vi "Send SetTemp Message.vi"(8 "error in (no error)":errorcluster, 10 "Cluster":cluster{"Temp":dbl, "Humid":dbl}, 11 "Execute":refnum<class "Execute.lvclass">) -> (0 "error out":errorcluster, 3 "Execute 2":refnum<class "Execute.lvclass">)   [LabVIEW 2018, in "QMH_Class.lvlib" / "TestManager.lvlib" / "SetTemp Message.lvclass"]
uses:
  SetTemp Message.lvclass
  Execute_class/Execute.lvclass
  E:/0 File/GITSync/DynoToolPlus/0 LabviewCode/0 Support/Message Queue_Class/Class/Message_class/InterfaceMessage/Interface Message.lvclass
  SetTemp Message.lvclass/SetTemp Message.ctl
  Execute_class/Execute.lvclass/Execute.ctl
  InterfaceMessage/Interface Message.lvclass
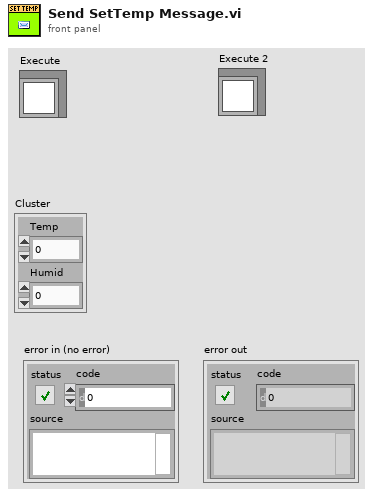
[diagram p1: front panel]
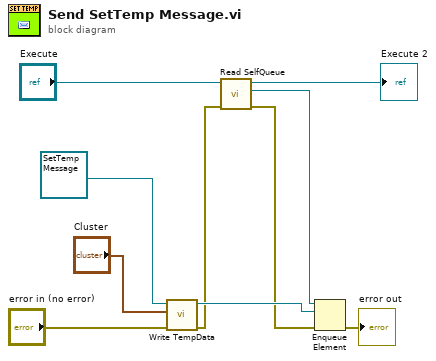
[diagram p0: block diagram]
diagram:
  n1 = call "Write TempData.vi"("error in (no error)"="error in (no error)", "TempData"="Cluster", "SetTemp Message"=refnum<class "SetTemp Message.lvclass"> refnum ("QMH_Class.lvlib:TestManager.lvlib:SetTemp Message.lvclass")) -> ("error out"=w2:errorcluster, "SetTemp Message"=w9:refnum<class "SetTemp Message.lvclass">)  [unwired: 7 in]
  n2 = call "Read SelfQueue.vi"("error in (no error)"=w2, "Execute"="Execute") -> ("error out"=w3:errorcluster, "SelfQueue"=w4:refnum<queue>, "Execute"=→"Execute 2":refnum<class "Execute.lvclass">)  [unwired: 7 in]
  n3 = Enqueue Element(queue=w4, element=w9, error in (no error)=w3) -> (error out=→"error out":errorcluster)  [unwired: 1 in, 2 out]
